vi "register subscriber.vi"(8 "error in":errorcluster {"code" format="Error %.0f"}, 10 "NATS Subscription":refnum<class "NATS Subscription.lvclass">, 11 "NATS Client in":refnum<class "NATS Client.lvclass">) -> (0 "error out":errorcluster {"code" format="Error %.0f"}, 3 "NATS Client out":refnum<class "NATS Client.lvclass">)   [LabVIEW 2024, in "NATS Client.lvlib" / "NATS Client.lvclass"]
uses:
  NATS Client.lvclass
  NATS Subscription/NATS Subscription.lvclass
  subscription queue.ctl
  subscription actions.ctl
  NATS Client.lvclass/NATS Client.ctl
  get subscriptions queue.vi
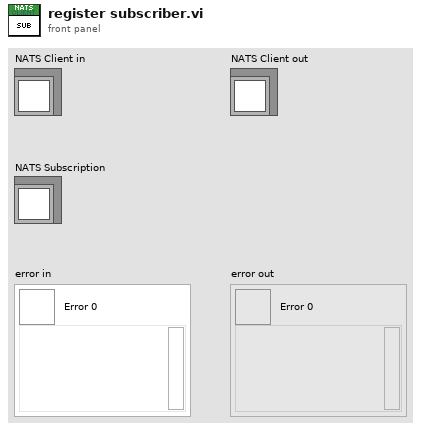
[diagram p1: front panel]
types:
  T1 = typedef "NATS Client.lvlib/NATS Client.lvclass/subscription actions.ctl" = enum16{"sub", "unsub"}
  T2 = typedef "NATS Client.lvlib/NATS Client.lvclass/subscription queue.ctl" = cluster{"action":T1, "subscription":refnum<class "NATS Subscription.lvclass">}
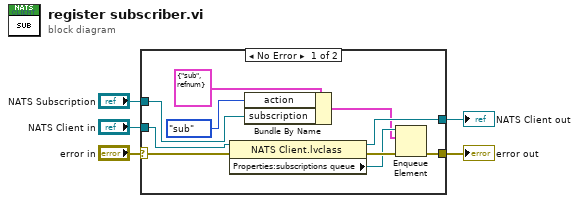
[diagram p0: block diagram]
diagram:
  n1 = case shown="No Error" "error in" {
    selector: "error in" -> [w15 w17]
    tunnel: [w14 w17] -> w4
    tunnel: [w11 w16] -> w2
    tunnel: "NATS Client in" -> [w10 w16]
    tunnel: "NATS Subscription" -> [w6 _]
    frame No Error {
      n2 = property class="NATS Client.lvclass"(reference=w10, error in=w15) -> (reference out=w11:refnum<class "NATS Client.lvclass">, error out=w13:errorcluster, "Properties:subscriptions queue"=w12:refnum<queue>)
      n3 = Bundle By Name(cluster=T2 {"action"=enum."sub", "subscription"=refnum} ("subscription queue"), "action"=subscription_actions."sub", "subscription"=w6) -> (w8:T2)
      n4 = Enqueue Element(queue=w12, element=w8, error in (no error)=w13) -> (error out=w14:errorcluster)  [unwired: 1 in, 2 out]
    }
    frame Error {
    }
  }
  "error out" <- w4
  "NATS Client out" <- w2
